vi "Sim System Server Set Battery Voltage.vi"(8 "error in (no error)":errorcluster, 11 "level":dbl) -> (0 "error out":errorcluster)   [LabVIEW 2026, in "MrcLib.lvlib"]
doc: "Set the battery voltage for your simulated robot."
uses:
  MrcLib.lvlib
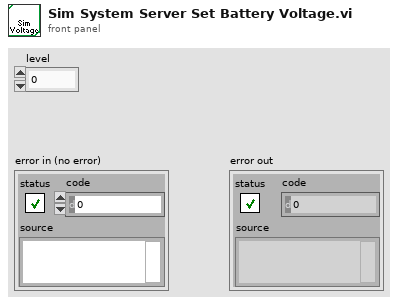
[diagram p1: front panel]
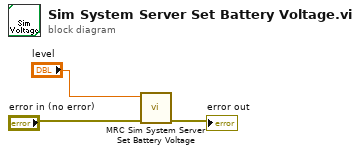
[diagram p0: block diagram]
diagram:
  n1 = call "MRC Sim System Server Set Battery Voltage.vi"("error in (no error)"="error in (no error)", "level"="level") -> ("error out"=→"error out":errorcluster)  [unwired: 9 in]
